vi "sv_Synchronize DSA Tasks.vi"(0 "master task in":refnum<k21>, 1 "action":enum16{"Synchronize", "Retrigger Start"}(ring), 5 "slave task in":refnum<k21>, 11 "error in (no error)":errorcluster) -> (4 "master task out":refnum<k21>, 6 "slave task out":refnum<k21>, 15 "error out":errorcluster)   [LabVIEW 2017]
doc: "Use this VI to sychronize DSA devices for stimulus-response measurements. Connect the master task input to the analog input task (measures wrap-back and response signals). Connect the slave task input to the analog output task (provides dynamic excitation signal)."
uses:
  <vilib>/DAQmx/configure/trigger.llb/DAQmx Start Trigger (Digital Edge).vi
  <resource>/objmgr/daqmx.rc
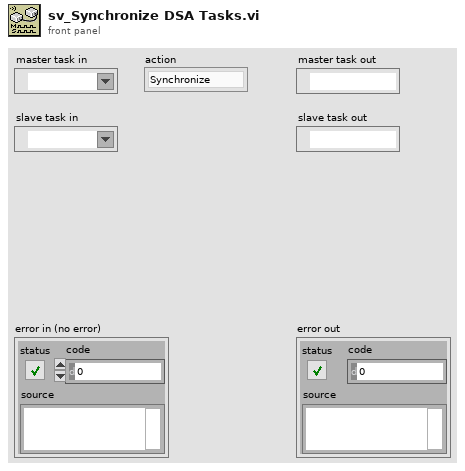
[diagram p1: front panel]
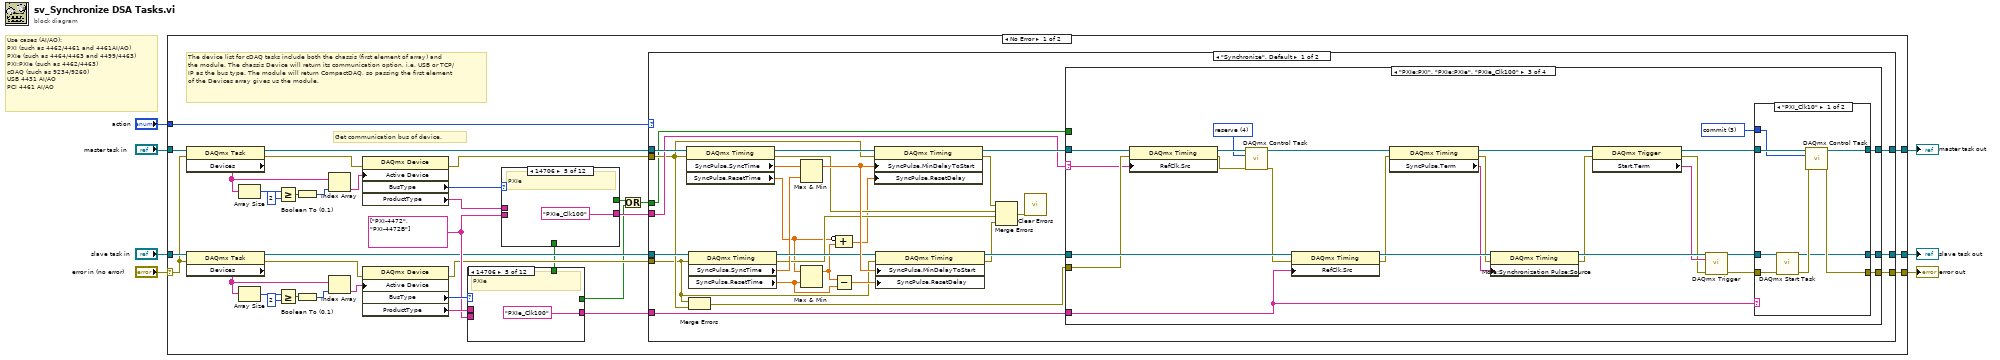
[diagram p0: block diagram]
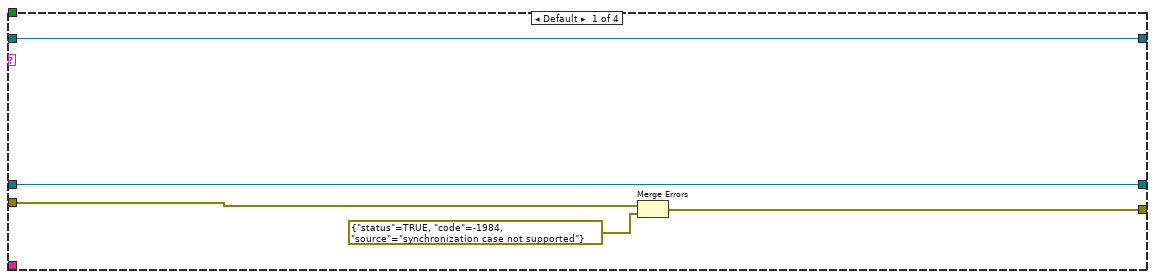
[diagram p2: hidden frame]
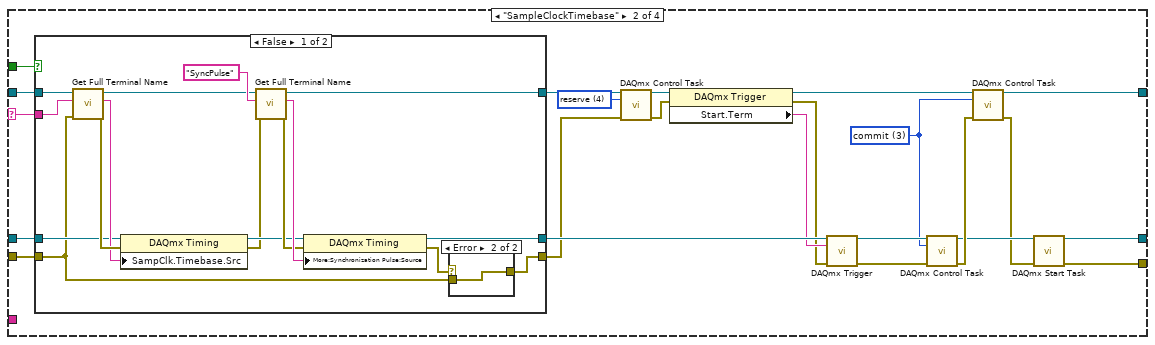
[diagram p3: hidden frame]
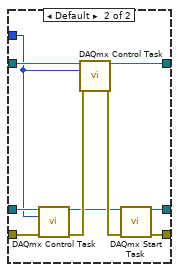
[diagram p6: hidden frame]
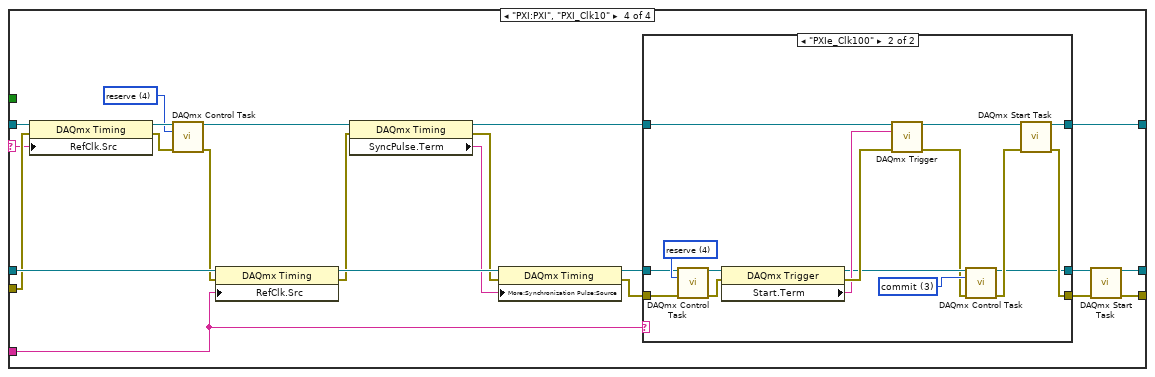
[diagram p7: hidden frame]
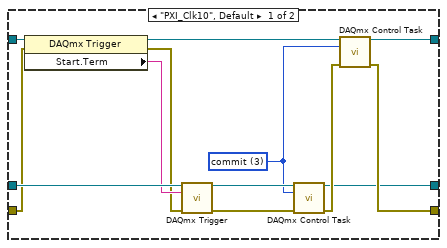
[diagram p8: hidden frame]
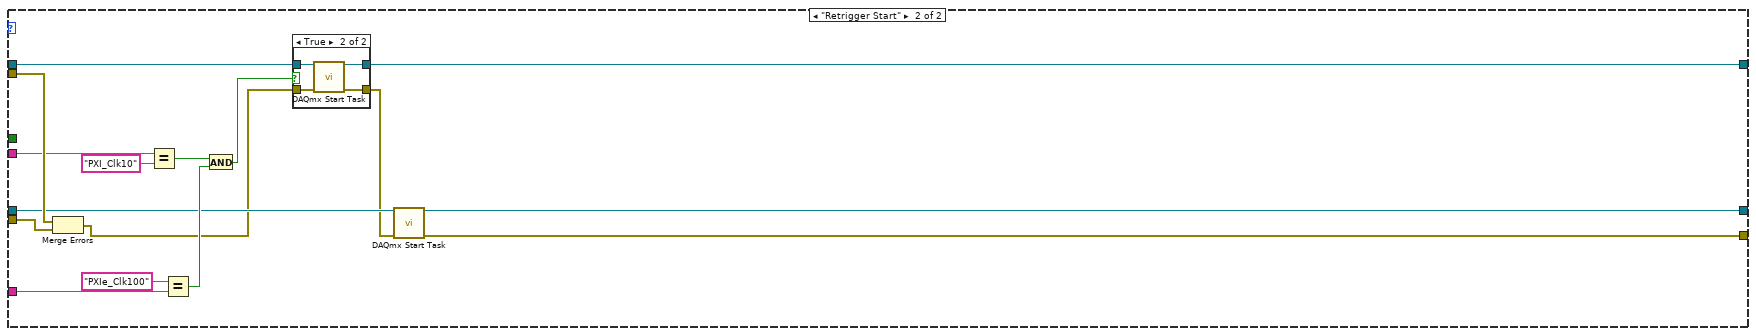
[diagram p9: hidden frame]
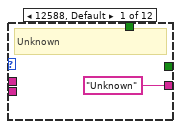
[diagram p11: hidden frame]
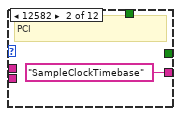
[diagram p12: hidden frame]
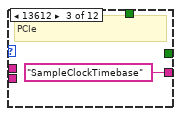
[diagram p13: hidden frame]
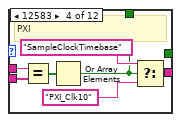
[diagram p14: hidden frame]
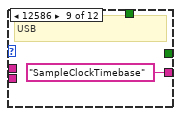
[diagram p18: hidden frame]
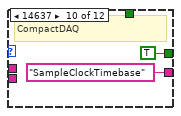
[diagram p19: hidden frame]
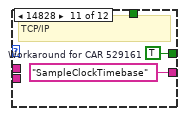
[diagram p20: hidden frame]
diagram:
  # "Use cases (AI/AO):\nPXI (such as 4462/4461 and 4461AI/AO)\nPXIe (such as 4464/4463 and 4499/4463)\nPXI:PXIe (such as 4462/4463)\ncDAQ (such as 9234/9260)\nUSB 4431 AI/AO\nPCI 4461 AI/AO"
  n1 = case shown="No Error" "error in (no error)" {
    selector: "error in (no error)" -> [w23 w274]
    tunnel: [w43 w272] -> w7
    tunnel: [w19 w273] -> w6
    tunnel: "slave task in" -> [w25 w273]
    tunnel: "master task in" -> [w24 w272]
    tunnel: [w18 w274] -> w3
    tunnel: "action" -> [w12 _]
    frame No Error {
      w26 = string[] ["PXI-4472", "PXI-4472B"]
      # "Get communication bus of device."
      # "The device list for cDAQ tasks include both the chassis (first element of array) and the module. The chassis Device will return its communication option, i.e. USB or TCP/IP as the bus type. The module will return CompactDAQ, so passing the first element of the Devices array gives us the module."
      n2 = property class="DAQmx Task"(reference=w24, error in=w23) -> (reference out=w17:refnum<k21>, error out=w22:errorcluster, "Devices"=w40:tag[])
      n3 = property class="DAQmx Task"(reference=w25, error in=w23) -> (reference out=w16:refnum<k21>, error out=w21:errorcluster, "Devices"=w32:tag[])
      n4 = Array Size(array=w40) -> (size(s)=w39:i32)
      n5 = Array Size(array=w32) -> (size(s)=w33:i32)
      n6 = Greater Or Equal?(x=w39, y=2 ("index")) -> (x >= y?=w37:bool)
      n7 = Greater Or Equal?(x=w33, y=2 ("index")) -> (x >= y?=w35:bool)
      n8 = Boolean To (0,1)(Boolean=w37) -> (0, 1=w36:i16)
      n9 = Boolean To (0,1)(Boolean=w35) -> (0, 1=w31:i16)
      n10 = Index Array(array=w40, index=w36) -> (element=w42:tag)
      n11 = Index Array(array=w32, index=w31) -> (element=w41:tag)
      n12 = property class="DAQmx Device"(error in=w22, "Active Device"=w42) -> (error out=w13:errorcluster, "BusType"=w30:i32, "ProductType"=w29:string)  [unwired: 1 in, 1 out]
      n13 = property class="DAQmx Device"(error in=w21, "Active Device"=w41) -> (error out=w14:errorcluster, "BusType"=w27:i32, "ProductType"=w28:string)  [unwired: 1 in, 1 out]
      n14 = case shown="14706" w27 {
        tunnel: ["Unknown" ("x") "SampleClockTimebase" ("x") "SampleClockTimebase" ("x") w243 "PXIe_Clk100" ("x") _ _ _ "SampleClockTimebase" ("x") "SampleClockTimebase" ("x") "SampleClockTimebase" ("x") _] -> w20
        tunnel: w28 -> [_ _ _ w247 _ _ _ _ _ _ _ _]
        tunnel: w26 -> [_ _ _ w246 _ _ _ _ _ _ _ _]
        tunnel: [_ _ _ w241 _ _ _ _ _ _ _ _] -> w11
        tunnel: [_ _ _ _ _ _ _ _ _ TRUE w252 _] -> w9
        frame 12588, Default {
          # "Unknown"
        }
        frame 12582 {
          # "PCI"
        }
        frame 13612 {
          # "PCIe"
        }
        frame 12583 {
          # "PXI"
          n15 = Equal?(x=w247, y=w246) -> (x = y?=w245:bool[])
          n16 = Or Array Elements(Boolean array=w245) -> (logical OR=w241:bool)
          n17 = Select(t="SampleClockTimebase" ("x"), s=w241, f="PXI_Clk10" ("x")) -> (s? t:f=w243:string)
        }
        frame 14706 {
          # "PXIe"
        }
        frame 12584 {
          # "SCXI"
        }
        frame 14707 {
          # "SCC"
        }
        frame 12585 {
          # "PCCard"
        }
        frame 12586 {
          # "USB"
        }
        frame 14637 {
          # "CompactDAQ"
        }
        frame 14828 {
          w252 = TRUE  # Workaround for CAR 529161
          # "TCP/IP"
        }
        frame 15870 {
          # "SwitchBlock"
        }
      }
      n18 = case shown="14706" w30 {
        tunnel: ["Unknown" ("x") "SampleClockTimebase" ("x") "SampleClockTimebase" ("x") w261 "PXIe_Clk100" ("x") _ _ _ "SampleClockTimebase" ("x") "SampleClockTimebase" ("x") "SampleClockTimebase" ("x") _] -> w15
        tunnel: w29 -> [_ _ _ w265 _ _ _ _ _ _ _ _]
        tunnel: w26 -> [_ _ _ w264 _ _ _ _ _ _ _ _]
        tunnel: w11 -> [_ _ _ w257 _ _ _ _ _ _ _ _]
        tunnel: [_ _ _ _ _ _ _ _ _ TRUE TRUE _] -> w10
        frame 12588, Default {
          # "Unknown"
        }
        frame 12582 {
          # "PCI"
        }
        frame 13612 {
          # "PCIe"
        }
        frame 12583 {
          # "PXI"
          n19 = Equal?(x=w265, y=w264) -> (x = y?=w263:bool[])
          n20 = Or Array Elements(Boolean array=w263) -> (logical OR=w259:bool)
          n21 = Or(x=w259, y=w257) -> (x .or. y?=w258:bool)
          n22 = Select(t="SampleClockTimebase" ("x"), s=w258, f="PXI_Clk10" ("x")) -> (s? t:f=w261:string)
        }
        frame 14706 {
          # "PXIe"
        }
        frame 12584 {
          # "SCXI"
        }
        frame 14707 {
          # "SCC"
        }
        frame 12585 {
          # "PCCard"
        }
        frame 12586 {
          # "USB"
        }
        frame 14637 {
          # "CompactDAQ"
        }
        frame 14828 {
          # "TCP/IP"
        }
        frame 15870 {
          # "SwitchBlock"
        }
      }
      n23 = Or(x=w10, y=w9) -> (x .or. y?=w8:bool)
      n24 = case shown="\"Synchronize\", Default" w12 {
        tunnel: [w52 w219] -> w43
        tunnel: w20 -> [w71 w226]
        tunnel: [w51 w221] -> w19
        tunnel: [w50 w222] -> w18
        tunnel: w17 -> [w64 w220]
        tunnel: w16 -> [w61 w223]
        tunnel: w15 -> [w58 w228]
        tunnel: w14 -> [w45 w230]
        tunnel: w13 -> [w46 w231]
        tunnel: w8 -> [w44 _]
        frame "Synchronize", Default {
          n25 = property class="DAQmx Timing"(reference=w64, error in=w46) -> (reference out=w67:refnum<k21>, error out=w60:errorcluster, "SyncPulse.SyncTime"=w65:dbl, "SyncPulse.ResetTime"=w53:dbl)
          n26 = property class="DAQmx Timing"(reference=w61, error in=w45) -> (reference out=w68:refnum<k21>, error out=w59:errorcluster, "SyncPulse.SyncTime"=w66:dbl, "SyncPulse.ResetTime"=w54:dbl)
          n27 = Merge Errors(w45, w46) -> (w70:errorcluster)
          n28 = Max & Min(x=w65, y=w66) -> (max(x,y)=w69:dbl)  [unwired: 1 out]
          n29 = Max & Min(x=w53, y=w54) -> (max(x,y)=w62:dbl)  [unwired: 1 out]
          n30 = Subtract(x=w62, y=w54) -> (x-y=w55:dbl)
          n31 = Compound Arithmetic op=ADD(invert w53, w62) -> (w56:dbl)
          n32 = property class="DAQmx Timing"(reference=w67, error in=w46, "SyncPulse.MinDelayToStart"=w69, "SyncPulse.ResetDelay"=w56) -> (reference out=w63:refnum<k21>, error out=w49:errorcluster)
          n33 = property class="DAQmx Timing"(reference=w68, error in=w45, "SyncPulse.MinDelayToStart"=w69, "SyncPulse.ResetDelay"=w55) -> (reference out=w57:refnum<k21>, error out=w48:errorcluster)
          n34 = Merge Errors(w49, w60, w59, w48) -> (w47:errorcluster)
          n35 = call <vilib>:"Clear Errors.vi"("error in (no error)"=w47) -> ()  [unwired: 5 in, 2 out]
          n36 = case shown="\"PXIe:PXI\", \"PXIe:PXIe\", \"PXIe_Clk100\"" w58 {
            selector: w58 -> [_ w93 w131 w172]
            tunnel: [w76 w90 w127 w176] -> w52
            tunnel: [w75 w83 w123 w166] -> w51
            tunnel: [w73 w84 w124 w165] -> w50
            tunnel: w63 -> [w76 w94 w134 w175]
            tunnel: w57 -> [w75 w96 w133 w174]
            tunnel: w70 -> [w72 w95 w132 w173]
            tunnel: w71 -> [_ _ w122 w171]
            tunnel: w44 -> [_ w82 _ _]
            frame Default {
              n37 = Merge Errors(w72, errorcluster {"status"=TRUE, "code"=-1984, "source"="synchronization case not supported"} ("error out")) -> (w73:errorcluster)
            }
            frame "SampleClockTimebase" {
              w77 = 4 items=["verify"=2, "reserve"=4, "commit"=3, "unreserve"=5, "abort"=6] ("action")
              w87 = 3 items=["verify"=2, "reserve"=4, "commit"=3, "unreserve"=5, "abort"=6] ("action")
              n38 = case shown="False" w82 {
                tunnel: [w115 w119] -> w99
                tunnel: [w112 w120] -> w78
                tunnel: w96 -> [w107 w119]
                tunnel: w95 -> [w100 w118]
                tunnel: w94 -> [w106 w120]
                tunnel: w93 -> [w104 _]
                tunnel: [w101 w118] -> w81
                frame False {
                  n39 = call "Get Full Terminal Name.vi"("error in"=w100, "Local Terminal Name"=w104, "task/channels in"=w106) -> ("error out"=w110:errorcluster, "Terminal Name with Device Prefix"=w109:tag, "task out"=w105:refnum<k21>)  [unwired: 6 in]
                  n40 = property class="DAQmx Timing"(reference=w107, error in=w110, "SampClk.Timebase.Src"=w109) -> (reference out=w108:refnum<k21>, error out=w103:errorcluster)
                  n41 = call "Get Full Terminal Name.vi"("error in"=w103, "Local Terminal Name"="SyncPulse", "task/channels in"=w105) -> ("error out"=w111:errorcluster, "Terminal Name with Device Prefix"=w114:tag, "task out"=w112:refnum<k21>)  [unwired: 6 in]
                  n42 = property class="DAQmx Timing"(reference=w108, error in=w111, "More:Synchronization Pulse:Source"=w114) -> (reference out=w115:refnum<k21>, error out=w102:errorcluster)
                  n43 = case shown="Error" w102 {
                    selector: w102 -> [w116 _]
                    tunnel: w100 -> [_ w117]
                    tunnel: [w116 w117] -> w101
                    frame No Error {
                    }
                    frame Error {
                    }
                  }
                }
                frame True {
                }
              }
              n44 = call <vilib>:"DAQmx Control Task.vi"("task/channels in"=w78, "action"=w77, "error in"=w81) -> ("task out"=w79:refnum<k21>, "error out"=w80:errorcluster)  [unwired: 11 in]
              n45 = property class="DAQmx Trigger"(reference=w79, error in=w80) -> (reference out=w91:refnum<k21>, error out=w97:errorcluster, "Start.Term"=w98:tag)
              n46 = call-poly <vilib>:"DAQmx Trigger.vi"("task/channels in"=w99, "source"=w98, "error in"=w97) -> ("task out"=w88:refnum<k21>, "error out"=w89:errorcluster)  [unwired: 11 in]
              n47 = call <vilib>:"DAQmx Control Task.vi"("task/channels in"=w88, "action"=w87, "error in"=w89) -> ("task out"=w86:refnum<k21>, "error out"=w92:errorcluster)  [unwired: 11 in]
              n48 = call <vilib>:"DAQmx Control Task.vi"("task/channels in"=w91, "action"=w87, "error in"=w92) -> ("task out"=w90:refnum<k21>, "error out"=w85:errorcluster)  [unwired: 11 in]
              n49 = call <vilib>:"DAQmx Start Task.vi"("task/channels in"=w86, "error in"=w85) -> ("task out"=w83:refnum<k21>, "error out"=w84:errorcluster)  [unwired: 12 in]
            }
            frame "PXIe:PXI", "PXIe:PXIe", "PXIe_Clk100" {
              w121 = 3 items=["verify"=2, "reserve"=4, "commit"=3, "unreserve"=5, "abort"=6] ("action")
              w140 = 4 items=["verify"=2, "reserve"=4, "commit"=3, "unreserve"=5, "abort"=6] ("action")
              n50 = property class="DAQmx Timing"(reference=w134, error in=w132, "RefClk.Src"=w131) -> (reference out=w141:refnum<k21>, error out=w126:errorcluster)
              n51 = call <vilib>:"DAQmx Control Task.vi"("task/channels in"=w141, "action"=w140, "error in"=w126) -> ("task out"=w138:refnum<k21>, "error out"=w125:errorcluster)  [unwired: 11 in]
              n52 = property class="DAQmx Timing"(reference=w133, error in=w125, "RefClk.Src"=w122) -> (reference out=w145:refnum<k21>, error out=w136:errorcluster)
              n53 = property class="DAQmx Timing"(reference=w138, error in=w136) -> (reference out=w139:refnum<k21>, error out=w135:errorcluster, "SyncPulse.Term"=w137:tag)
              n54 = property class="DAQmx Timing"(reference=w145, error in=w135, "More:Synchronization Pulse:Source"=w137) -> (reference out=w146:refnum<k21>, error out=w144:errorcluster)
              n55 = property class="DAQmx Trigger"(reference=w139, error in=w144) -> (reference out=w128:refnum<k21>, error out=w142:errorcluster, "Start.Term"=w143:tag)
              n56 = call-poly <vilib>:"DAQmx Trigger.vi"("task/channels in"=w146, "source"=w143, "error in"=w142) -> ("task out"=w130:refnum<k21>, "error out"=w129:errorcluster)  [unwired: 11 in]
              n57 = case shown="\"PXI_Clk10\"" w122 {
                tunnel: w130 -> [w152 w164]
                tunnel: w129 -> [w151 w163]
                tunnel: w128 -> [w154 w161]
                tunnel: [w153 w160] -> w127
                tunnel: [w149 w158] -> w124
                tunnel: [w148 w156] -> w123
                tunnel: w121 -> [w147 w155]
                frame "PXI_Clk10" {
                  n58 = call <vilib>:"DAQmx Start Task.vi"("task/channels in"=w152, "error in"=w151) -> ("task out"=w148:refnum<k21>, "error out"=w150:errorcluster)  [unwired: 12 in]
                  n59 = call <vilib>:"DAQmx Control Task.vi"("task/channels in"=w154, "action"=w147, "error in"=w150) -> ("task out"=w153:refnum<k21>, "error out"=w149:errorcluster)  [unwired: 11 in]
                }
                frame Default {
                  n60 = call <vilib>:"DAQmx Control Task.vi"("task/channels in"=w164, "action"=w155, "error in"=w163) -> ("task out"=w157:refnum<k21>, "error out"=w162:errorcluster)  [unwired: 11 in]
                  n61 = call <vilib>:"DAQmx Control Task.vi"("task/channels in"=w161, "action"=w155, "error in"=w162) -> ("task out"=w160:refnum<k21>, "error out"=w159:errorcluster)  [unwired: 11 in]
                  n62 = call <vilib>:"DAQmx Start Task.vi"("task/channels in"=w157, "error in"=w159) -> ("task out"=w156:refnum<k21>, "error out"=w158:errorcluster)  [unwired: 12 in]
                }
              }
            }
            frame "PXI:PXI", "PXI_Clk10" {
              w182 = 4 items=["verify"=2, "reserve"=4, "commit"=3, "unreserve"=5, "abort"=6] ("action")
              n63 = property class="DAQmx Timing"(reference=w175, error in=w173, "RefClk.Src"=w172) -> (reference out=w183:refnum<k21>, error out=w170:errorcluster)
              n64 = call <vilib>:"DAQmx Control Task.vi"("task/channels in"=w183, "action"=w182, "error in"=w170) -> ("task out"=w180:refnum<k21>, "error out"=w169:errorcluster)  [unwired: 11 in]
              n65 = property class="DAQmx Timing"(reference=w174, error in=w169, "RefClk.Src"=w171) -> (reference out=w185:refnum<k21>, error out=w178:errorcluster)
              n66 = property class="DAQmx Timing"(reference=w180, error in=w178) -> (reference out=w181:refnum<k21>, error out=w177:errorcluster, "SyncPulse.Term"=w179:tag)
              n67 = property class="DAQmx Timing"(reference=w185, error in=w177, "More:Synchronization Pulse:Source"=w179) -> (reference out=w186:refnum<k21>, error out=w184:errorcluster)
              n68 = case shown="\"PXIe_Clk100\"" w171 {
                tunnel: w186 -> [w199 w204]
                tunnel: w181 -> [w196 w206]
                tunnel: w184 -> [w195 w203]
                tunnel: [w187 w200] -> w168
                tunnel: [w190 w201] -> w167
                tunnel: [w189 w205] -> w176
                frame "PXI_Clk10", Default {
                  w192 = 3 items=["verify"=2, "reserve"=4, "commit"=3, "unreserve"=5, "abort"=6] ("action")
                  n69 = property class="DAQmx Trigger"(reference=w196, error in=w195) -> (reference out=w188:refnum<k21>, error out=w197:errorcluster, "Start.Term"=w198:tag)
                  n70 = call-poly <vilib>:"DAQmx Trigger.vi"("task/channels in"=w199, "source"=w198, "error in"=w197) -> ("task out"=w193:refnum<k21>, "error out"=w191:errorcluster)  [unwired: 11 in]
                  n71 = call <vilib>:"DAQmx Control Task.vi"("task/channels in"=w193, "action"=w192, "error in"=w191) -> ("task out"=w187:refnum<k21>, "error out"=w194:errorcluster)  [unwired: 11 in]
                  n72 = call <vilib>:"DAQmx Control Task.vi"("task/channels in"=w188, "action"=w192, "error in"=w194) -> ("task out"=w189:refnum<k21>, "error out"=w190:errorcluster)  [unwired: 11 in]
                }
                frame "PXIe_Clk100" {
                  w211 = 3 items=["verify"=2, "reserve"=4, "commit"=3, "unreserve"=5, "abort"=6] ("action")
                  w214 = 4 items=["verify"=2, "reserve"=4, "commit"=3, "unreserve"=5, "abort"=6] ("action")
                  n73 = call <vilib>:"DAQmx Control Task.vi"("task/channels in"=w204, "action"=w214, "error in"=w203) -> ("task out"=w215:refnum<k21>, "error out"=w202:errorcluster)  [unwired: 11 in]
                  n74 = property class="DAQmx Trigger"(reference=w215, error in=w202) -> (reference out=w210:refnum<k21>, error out=w213:errorcluster, "Start.Term"=w212:tag)
                  n75 = call-poly <vilib>:"DAQmx Trigger.vi"("task/channels in"=w206, "source"=w212, "error in"=w213) -> ("task out"=w207:refnum<k21>, "error out"=w209:errorcluster)  [unwired: 11 in]
                  n76 = call <vilib>:"DAQmx Control Task.vi"("task/channels in"=w210, "action"=w211, "error in"=w209) -> ("task out"=w200:refnum<k21>, "error out"=w208:errorcluster)  [unwired: 11 in]
                  n77 = call <vilib>:"DAQmx Start Task.vi"("task/channels in"=w207, "error in"=w208) -> ("task out"=w205:refnum<k21>, "error out"=w201:errorcluster)  [unwired: 12 in]
                }
              }
              n78 = call <vilib>:"DAQmx Start Task.vi"("task/channels in"=w168, "error in"=w167) -> ("task out"=w166:refnum<k21>, "error out"=w165:errorcluster)  [unwired: 12 in]
            }
          }
        }
        frame "Retrigger Start" {
          n79 = Merge Errors(w231, w230) -> (w217:errorcluster)
          n80 = Equal?(x=w228, y="PXI_Clk10" ("x")) -> (x = y?=w225:bool)
          n81 = Equal?(x="PXIe_Clk100", y=w226) -> (x = y?=w224:bool)
          n82 = And(x=w225, y=w224) -> (x .and. y?=w218:bool)
          n83 = case shown="True" w218 {
            tunnel: w220 -> [w233 w237]
            tunnel: [w233 w236] -> w219
            tunnel: w217 -> [w232 w235]
            tunnel: [w232 w234] -> w216
            frame False {
            }
            frame True {
              n84 = call <vilib>:"DAQmx Start Task.vi"("task/channels in"=w237, "error in"=w235) -> ("task out"=w236:refnum<k21>, "error out"=w234:errorcluster)  [unwired: 12 in]
            }
          }
          n85 = call <vilib>:"DAQmx Start Task.vi"("task/channels in"=w223, "error in"=w216) -> ("task out"=w221:refnum<k21>, "error out"=w222:errorcluster)  [unwired: 12 in]
        }
      }
    }
    frame Error {
    }
  }
  "error out" <- w3
  "master task out" <- w7
  "slave task out" <- w6
